vi "1710_模拟量输出.vi"() -> ()   [LabVIEW 2015]
uses:
  <userlib>/DAQNavi Polymorphic VI/create/DAQNavi Create Channel(AO-Voltage).vi
  <userlib>/DAQNavi Polymorphic VI/write/DAQNavi Write (Analog DBL 1Chan 1Samp).vi
panel:
  out "number of samples written per channel":u32
  in  "data":dbl
  out "error out":errorcluster
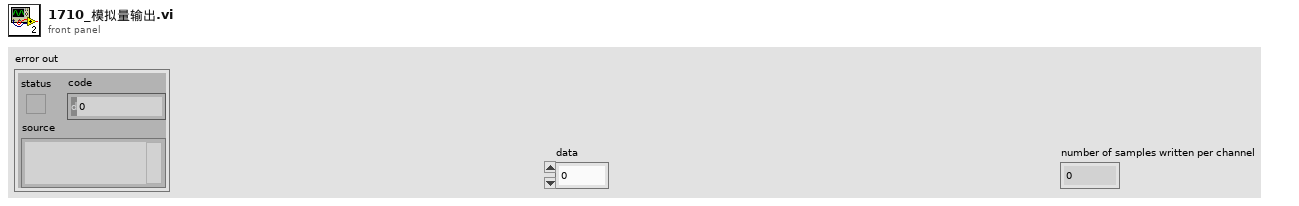
[diagram p1: front panel]
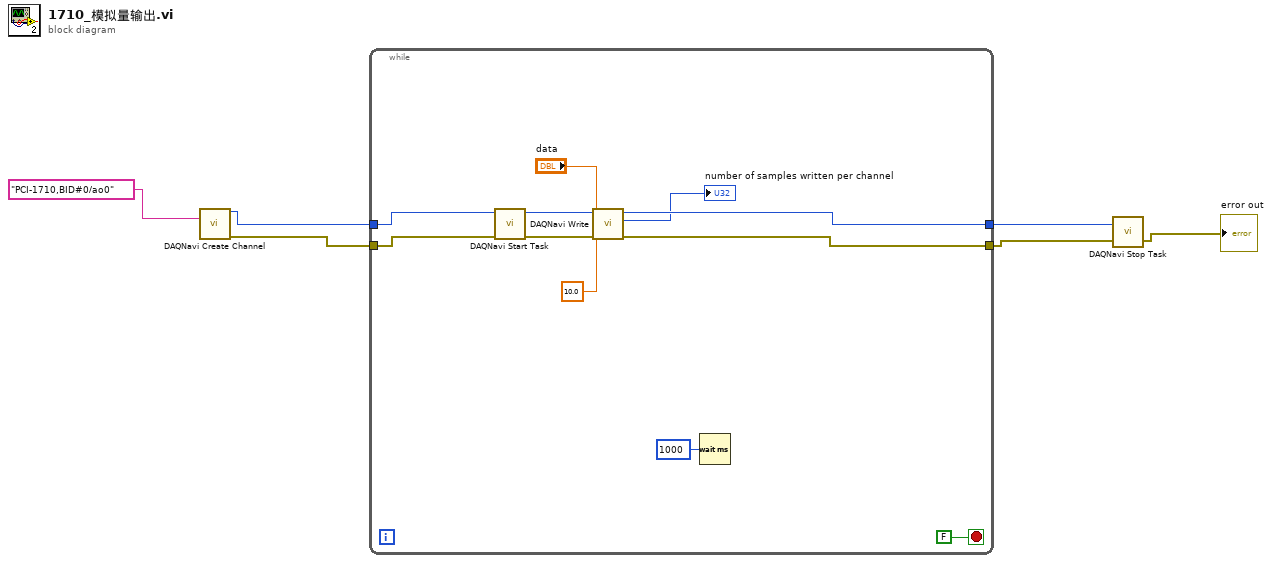
[diagram p0: block diagram]
diagram:
  n1 = call-poly <userlib>:"DAQNavi Create Channel.vi"("physical channels"="PCI-1710,BID#0/ao0") -> ("task out"=w5:i32, "error out"=w4:errorcluster)  [unwired: 13 in]
  n2 = while {
    tunnel: w5 -> [w17]
    tunnel: [w14] -> w3
    tunnel: w4 -> [w16]
    tunnel: [w13] -> w2
    stop <- FALSE stop-if-true
    n3 = call <userlib>:"DAQNavi Start Task.vi"("error in (no error)"=w16, "task in"=w17) -> ("error out"=w15:errorcluster, "task out"=w8:i32)  [unwired: 8 in]
    n4 = call-poly <userlib>:"DAQNavi Write.vi"("error in (no error)"=w15, "timeout"=10.0, "data"="data", "task in"=w8) -> ("error out"=w13:errorcluster, "number of samples written per channel"=→"number of samples written per channel":u32, "task out"=w14:i32)  [unwired: 5 in]
    n5 = Wait (ms)(milliseconds to wait=u32 1000 ("等待时间（毫秒）")) -> ()  [unwired: 1 out]
  }
  n6 = call <userlib>:"DAQNavi Stop Task.vi"("error in (no error)"=w2, "task in"=w3) -> ("error out"=→"error out":errorcluster)  [unwired: 1 out]
